vi "Load_from_Project.vi"(8 "error in (no error)":errorcluster, 9 "index":string, 10 "buildObject":T1, 11 "IB_SoftDependency in":refnum<class "IB_SoftDependency.lvclass">) -> (0 "error out":errorcluster, 1 "index out":string, 2 "buildObject out":T1, 3 "IB_SoftDependency out":refnum<class "IB_SoftDependency.lvclass">)   [LabVIEW 2020, in "IB_SoftDependency.lvclass"]
uses:
  <vilib>/AppBuilder/IB_Classes/SoftDependency/IB_SoftDependency.lvclass
  <vilib>/AppBuilder/IB_Classes/SoftDependency/IB_SoftDependency.lvclass/IB_SoftDependency.ctl
  <vilib>/AppBuilder/IB_RW_Project/IB_RW_Project_PropBag_Action.ctl
  <resource>/Framework/Providers/API/ItemRef.ctl
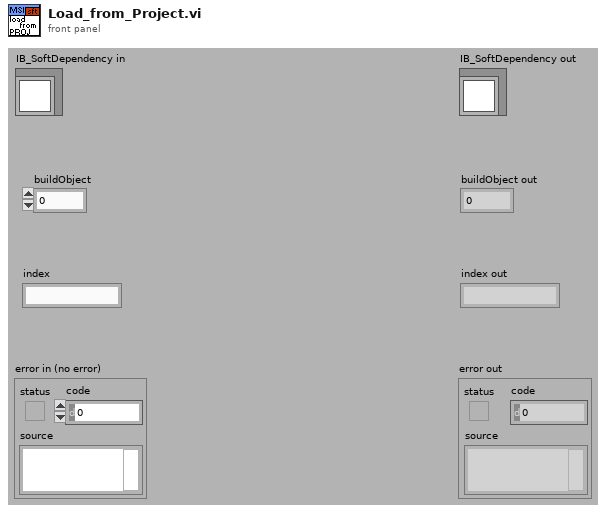
[diagram p1: front panel]
types:
  T1 = typedef "ItemRef.ctl" = u64
  T2 = typedef "IB_RW_Project_PropBag_Action.ctl" = enum16{"read", "write", "clear", "readPrevious", "writePrevious", "clearPrevious"}
  T3 = typedef "IB_RW_Project_SoftDep_Data.ctl" = cluster{"ProductName":string, "UpgradeCode":string, "exclude?":bool}
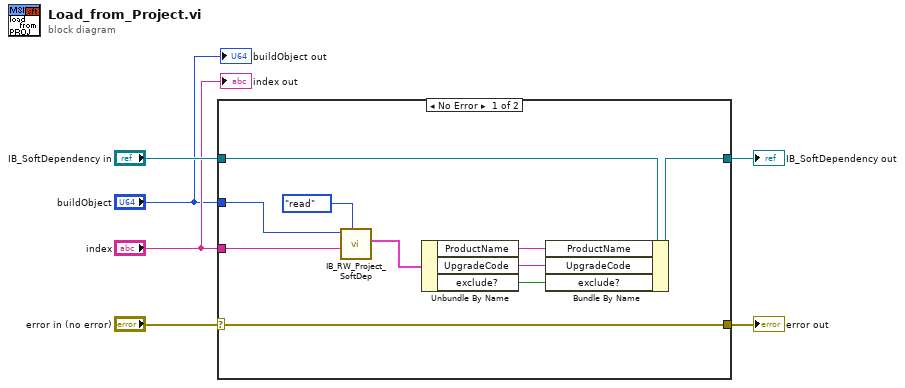
[diagram p0: block diagram]
diagram:
  n1 = case shown="No Error" "error in (no error)" {
    selector: "error in (no error)" -> [w16 w18]
    tunnel: [w16 w18] -> w5
    tunnel: [w9 w17] -> w3
    tunnel: "IB_SoftDependency in" -> [w10 w17]
    tunnel: "buildObject" -> [w12 _]
    tunnel: "index" -> [w11 _]
    frame No Error {
      n2 = call <vilib>:"IB_RW_Project_SoftDep.vi"("action"=IB_RW_Project_PropBag_Action."read", "index in"=w11, "buildObject"=w12) -> ("dataSource out"=w14:T3)  [unwired: 2 in, 6 out]
      n3 = Unbundle By Name(w14) -> ("ProductName"=w15:string, "UpgradeCode"=w8:string, "exclude?"=w7:bool)
      n4 = Bundle By Name(cluster=w10, "ProductName"=w15, "UpgradeCode"=w8, "exclude?"=w7) -> (w9:refnum<class "IB_SoftDependency.lvclass">)
    }
    frame Error {
    }
  }
  "error out" <- w5
  "IB_SoftDependency out" <- w3
  "buildObject out" <- "buildObject"
  "index out" <- "index"
